vi "ping.vi"(8 "error in":errorcluster, 9 "timeout (ms)":i32=1000, 10 "count":i32=1, 11 "host":string="127.0.0.1") -> (0 "error out":errorcluster, 2 "found?":bool, 3 "IP":string)   [LabVIEW 2013]
doc: "This VI allows you to ping a host and pass parameters to define the number of attempts and timeout. The default timeout is set to 1000 ms."
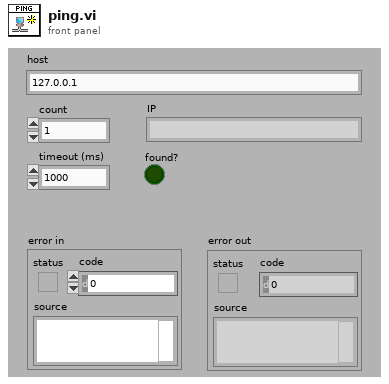
[diagram p1: front panel]
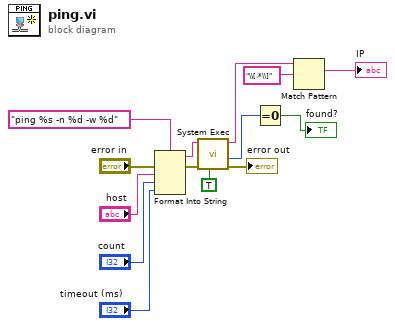
[diagram p0: block diagram]
diagram:
  n1 = Format Into String(format string="ping %s -n %d -w %d", error in="error in", "host", "count", "timeout (ms)") -> (resulting string=w7:string, error out=w13:errorcluster)  [unwired: 1 in]
  n2 = call <vilib>:"System Exec.vi"("run minimized? (F)"=TRUE, "error in (no error)"=w13, "command line"=w7) -> ("error out"=→"error out":errorcluster, "return code"=w6:i32, "standard output"=w4:string)  [unwired: 5 in, 1 out]
  n3 = Equal To 0?(x=w6) -> (x = 0?=→"found?":bool)
  n4 = Match Pattern(string=w4, regular expression="\\[.*\\]") -> (match substring=→"IP":string)  [unwired: 1 in, 3 out]
